vi "OLD get last camera data.vi"(7 "Now":timestamp, 8 "life time":dbl, 9 "camera_id":u32, 11 "Detection Frame In":T2) -> ()   [LabVIEW 2016]
uses:
  SSL Detection Frame.ctl
  SSL Detection Robot.ctl
  SSL Detection Ball.ctl
panel:
  out "team estimator":T1[](array[typedef]) {"height" format="%+4.3f"; "pixel_y" format="%+4.3f"; "pixel_x" format="%+4.3f"; "orientation" format="%+4.3f"; "y" format="%+4.3f"; "confidence" format="%4.3f"; "x" format="%+4.3f"}
  # "recebe os dados de uma câmera, armazena apenas o mais recente"
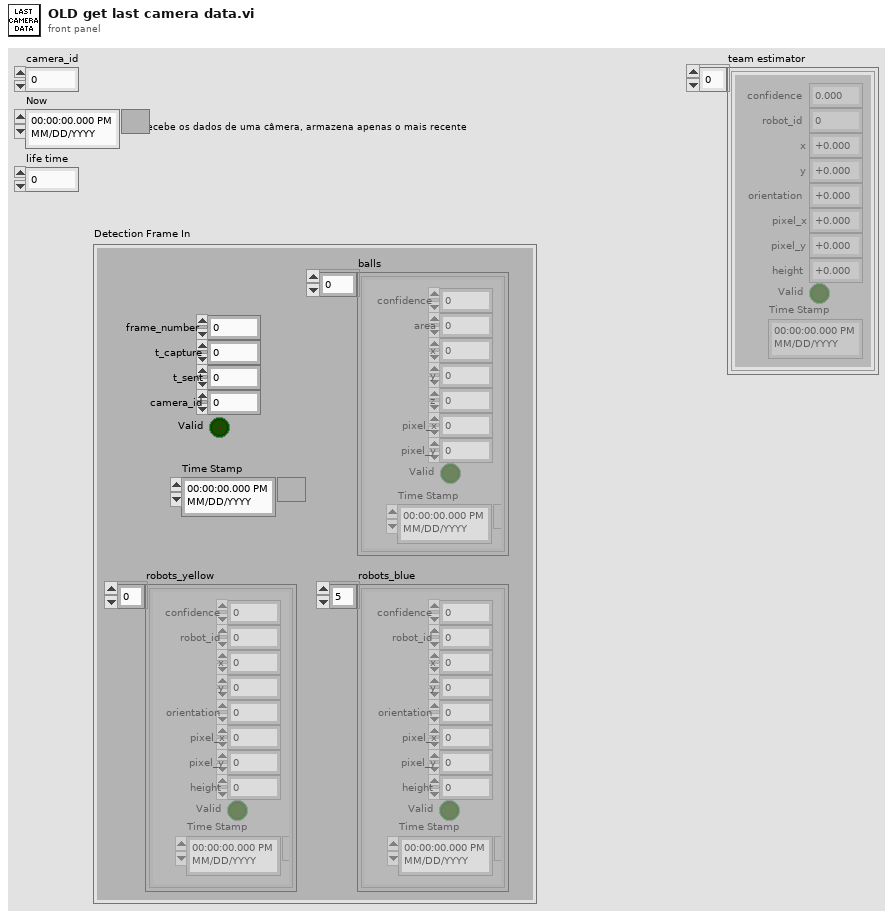
[diagram p1: front panel]
types:
  T1 = typedef "SSL Detection Robot.ctl" = cluster{"x":dbl, "robot_id":u32, "confidence":sgl, "y":sgl, "orientation":sgl, "pixel_x":sgl, "pixel_y":sgl, "height":sgl, "Valid":bool, "Time Stamp":timestamp}
  T2 = typedef "SSL Detection Frame.ctl" = cluster{"frame_number":u32, "t_capture":dbl, "t_sent":dbl, "camera_id":u32, "robots_yellow":T1[], "robots_blue":T1[], "balls":T3[], "Valid":bool, "Time Stamp":timestamp}
  T3 = typedef "SSL Detection Ball.ctl" = cluster{"x":sgl, "area":u32, "confidence":sgl, "y":sgl, "z":sgl, "pixel_x":sgl, "pixel_y":sgl, "Valid":bool, "Time Stamp":timestamp}
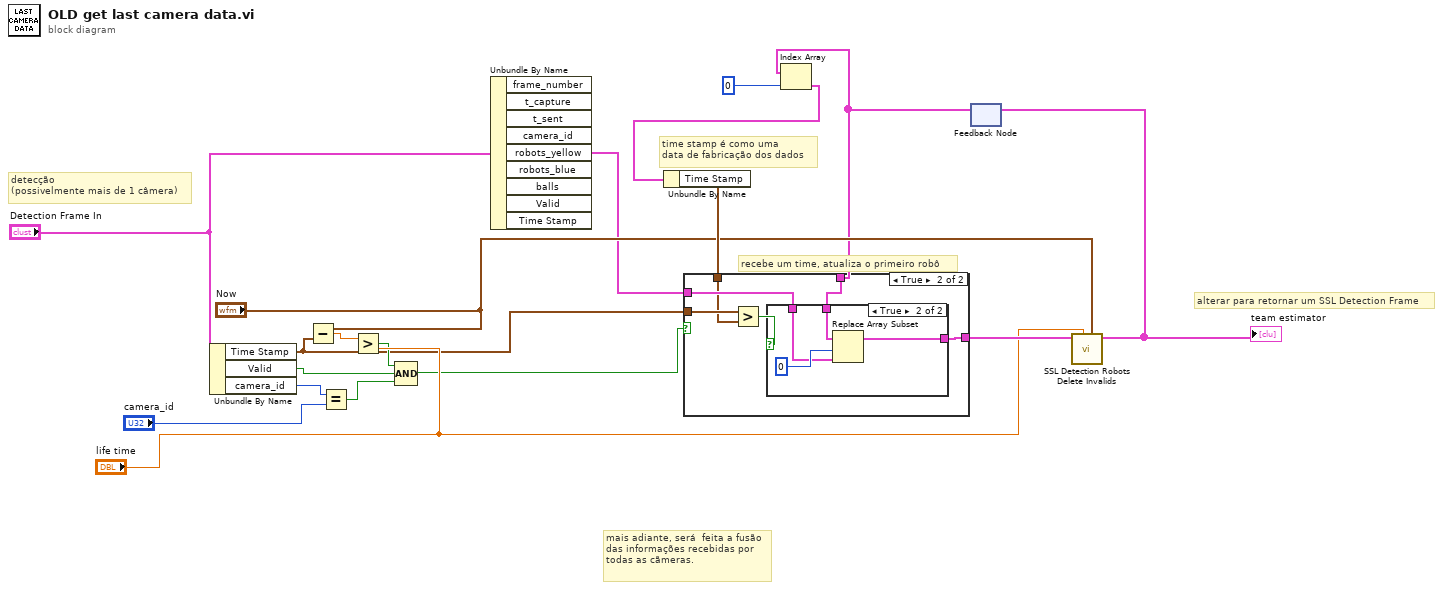
[diagram p0: block diagram]
diagram:
  # "alterar para retornar um SSL Detection Frame"
  # "recebe um time, atualiza o primeiro robô"
  # "time stamp é como uma\ndata de fabricação dos dados"
  # "mais adiante, será  feita a fusão das informações recebidas por todas as cãmeras."
  # "detecção\n(possivelmente mais de 1 câmera)"
  n1 = Unbundle By Name("Detection Frame In") -> ("Time Stamp"=w7:timestamp, "Valid"=w10:bool, "camera_id"=w12:u32)
  n2 = Subtract(x="Now", y=w7) -> (x-y=w9:dbl)
  n3 = Equal?(x=w12, y="camera_id") -> (x = y?=w11:bool)
  n4 = Greater?(x=w9, y="life time") -> (0:w8:bool)
  n5 = Compound Arithmetic op=AND(w8, w10, w11) -> (w6:bool)
  n6 = Unbundle By Name("Detection Frame In") -> ("robots_yellow"=w5:T1[])  [unwired: 8 out]
  n7 = feedback #1() -> (w4:T1[])  [unwired: 1 in]
  n8 = Index Array(array=w4, index=0) -> (element=w2:T1)
  n9 = Unbundle By Name(w2) -> ("Time Stamp"=w16:timestamp)
  n10 = case shown="True" w6 {
    tunnel: w16 -> [_ w20]
    tunnel: w7 -> [_ w25]
    tunnel: w5 -> [_ w23]
    tunnel: [w19 w22] -> w15
    tunnel: w4 -> [w19 w21]
    frame False {
    }
    frame True {
      n11 = Greater?(x=w25, y=w20) -> (0:w24:bool)
      n12 = case shown="True" w24 {
        tunnel: w23 -> [_ w29]
        tunnel: [w26 w27] -> w22
        tunnel: w21 -> [w26 w28]
        frame False {
        }
        frame True {
          n13 = Replace Array Subset(array=w28, new element=w29, index=0) -> (w27:T1[])
        }
      }
    }
  }
  n14 = call "SSL Detection Robots Delete Invalids.vi"("Now"="Now", "Life Time"="life time", "Robots In"=w15) -> ("Robots Out"=w1:T1[])  [unwired: 8 in]
  "team estimator" <- w1
  n15 = feedback-in #1(w1) -> ()
